vi "Ping_Test.vi"(11 "IP Address":string) -> (0 "PASS?":bool)   [LabVIEW 2016]
panel:
  out "standard output":string
  out "standard error":string
  in  "error in (no error)":errorcluster
  out "error out":errorcluster
  out "Cmd":string
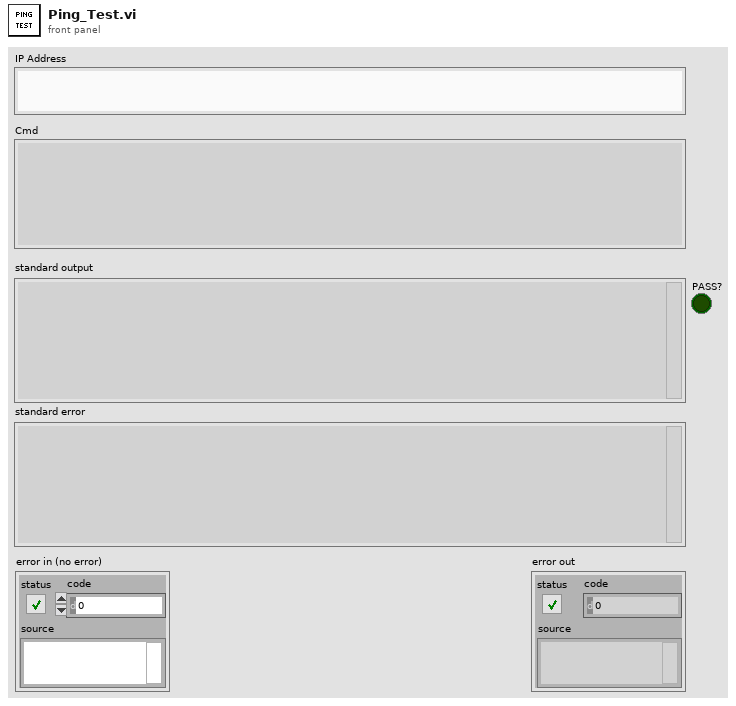
[diagram p1: front panel]
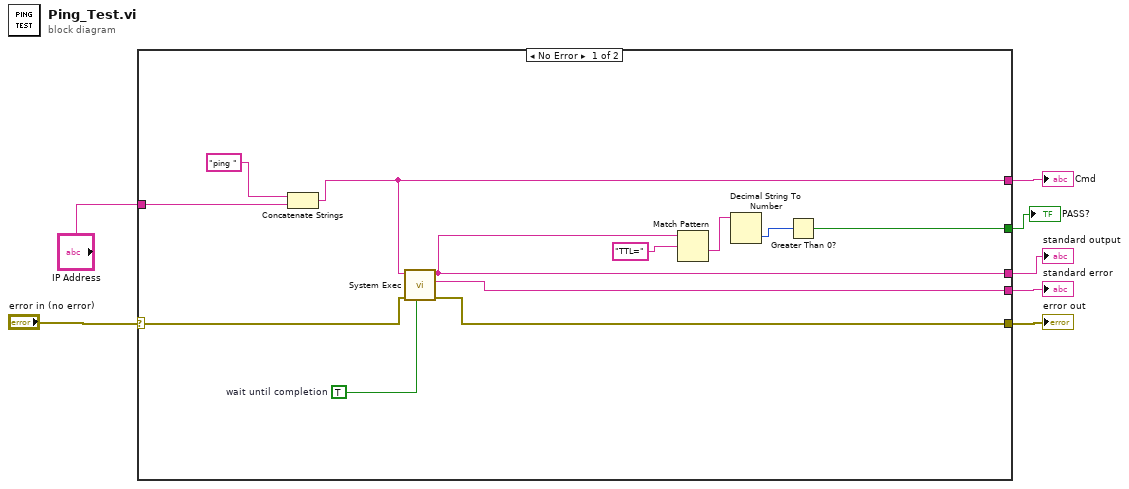
[diagram p0: block diagram]
diagram:
  n1 = case shown="No Error" "error in (no error)" {
    selector: "error in (no error)" -> [w16 w20]
    tunnel: [w19 _] -> w4
    tunnel: [w18 w20] -> w5
    tunnel: [w11 _] -> w7
    tunnel: [w12 _] -> w3
    tunnel: "IP Address" -> [w9 _]
    tunnel: [w8 _] -> w1
    frame No Error {
      w17 = TRUE  # wait until completion
      n2 = Concatenate Strings("ping " ("string"), w9) -> (w11:string)
      n3 = call <vilib>:"System Exec.vi"("run minimized? (F)"=w17, "error in (no error)"=w16, "command line"=w11) -> ("error out"=w18:errorcluster, "standard error"=w19:string, "standard output"=w8:string)  [unwired: 5 in, 1 out]
      n4 = Match Pattern(string=w8, regular expression="TTL=") -> (after substring=w14:string)  [unwired: 1 in, 3 out]
      n5 = Decimal String To Number(string=w14) -> (number=w13:i32)  [unwired: 2 in, 1 out]
      n6 = Greater Than 0?(x=w13) -> (x > 0?=w12:bool)
    }
    frame Error {
    }
  }
  "standard output" <- w1
  "standard error" <- w4
  "error out" <- w5
  "Cmd" <- w7
  "PASS?" <- w3
